vi "DriverStationData.vi"() -> (3 "DriverStation_Data":T1)   [LabVIEW 2017]
uses:
  DriverStation_TypeDef.ctl
  <vilib>/Rock Robotics/WPI/DriverStation/WPI_DriverStationAllianceInfo.ctl
  <vilib>/Rock Robotics/WPI/DriverStation/WPI_DriverStationPositionInfo.ctl
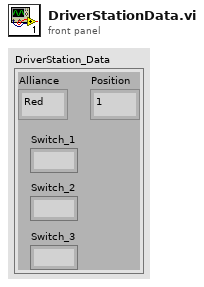
[diagram p1: front panel]
types:
  T1 = typedef "DriverStation_TypeDef.ctl" = cluster{"Alliance":T2, "Position":T3, "Switch_1":string, "Switch_2":string, "Switch_3":string}
  T2 = typedef "WPI_DriverStationAllianceInfo.ctl" = enum16{"Red", "Blue", "Invalid"}
  T3 = typedef "WPI_DriverStationPositionInfo.ctl" = enum16{"1", "2", "3"}
  T4 = cluster{"Alliance":T2, "Position":T3, "Game Specific Data":string, "Game Specific Data":string, "Game Specific Data":string}
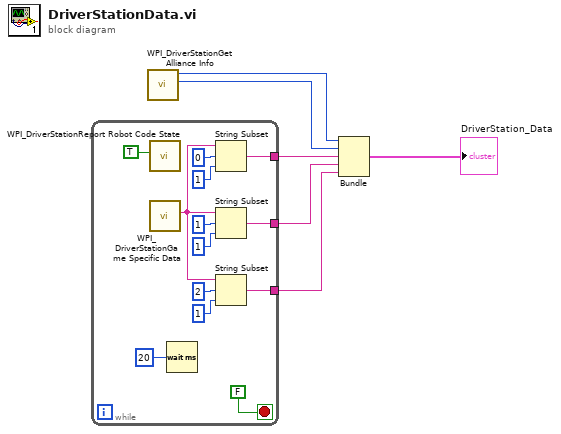
[diagram p0: block diagram]
diagram:
  n1 = while {
    tunnel: [w9] -> w3
    tunnel: [w8] -> w2
    tunnel: [w7] -> w1
    stop <- FALSE stop-if-true
    n2 = call <vilib>:"WPI_DriverStationReport Robot Code State.vi"("Autonomous"=TRUE) -> ()  [unwired: 10 in, 1 out]
    n3 = call <vilib>:"WPI_DriverStationGame Specific Data.vi"() -> ("Game Specific Data"=w10:string)  [unwired: 11 in]
    n4 = Wait (ms)(milliseconds to wait=u32 20) -> ()  [unwired: 1 out]
    n5 = String Subset(string=w10, offset (0)=0, length (rest)=1 ("length (rest)")) -> (substring=w9:string)
    n6 = String Subset(string=w10, offset (0)=1, length (rest)=1 ("length (rest)")) -> (substring=w8:string)
    n7 = String Subset(string=w10, offset (0)=2, length (rest)=1 ("length (rest)")) -> (substring=w7:string)
  }
  n8 = call <vilib>:"WPI_DriverStationGet Alliance Info.vi"() -> ("Position"=w5:T3, "Alliance"=w6:T2)  [unwired: 10 out]
  n9 = Bundle("Alliance"=w6, "Position"=w5, "Game Specific Data"=w3, "Game Specific Data"=w2, "Game Specific Data"=w1) -> (→"DriverStation_Data":T4)  [unwired: 1 in]
